vi "Get Initial FP Control Positions.vi"(8 "error in (no error)":errorcluster, 9 "Pane 2":refnum<vi>, 10 "Pane":refnum<vi>, 11 "Message Log in":refnum<class "Message Log.lvclass">) -> (0 "error out":errorcluster, 3 "Message Log out":refnum<class "Message Log.lvclass">)   [LabVIEW 2017, in "Message Log.lvclass"]
doc: "Get the initial positons of resizable front panel elements"
uses:
  Message Log.lvclass
  Message Log.lvclass/Message Log.ctl
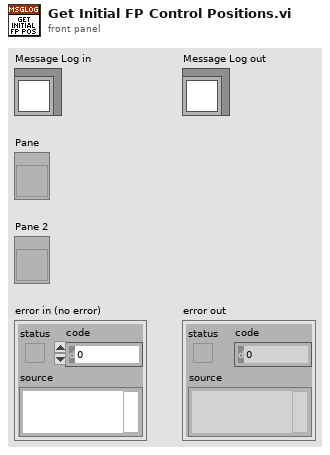
[diagram p1: front panel]
types:
  T1 = typedef "LVBoundsTypeDef.ctl" = cluster{"Width":u32, "Height":u32}
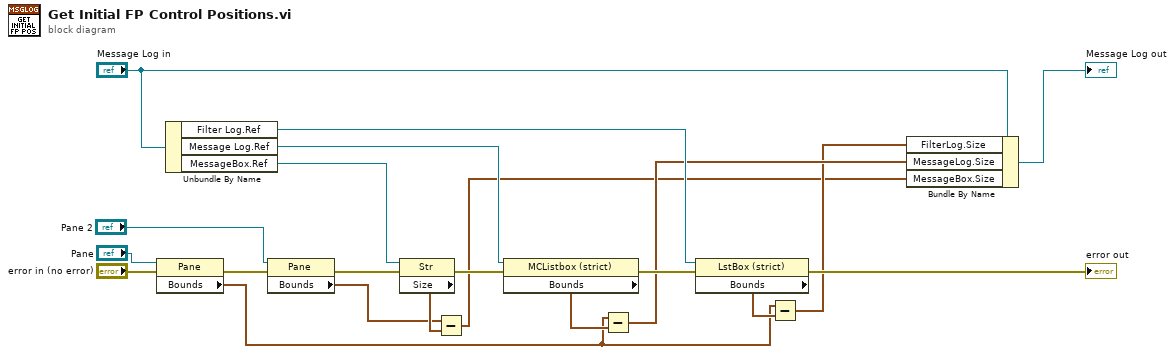
[diagram p0: block diagram]
diagram:
  n1 = property class="Pane"(reference="Pane", error in="error in (no error)") -> (error out=w14:errorcluster, "Bounds"=w1:T1)  [unwired: 1 out]
  n2 = Unbundle By Name("Message Log in") -> ("Filter Log.Ref"=w12:refnum<vi>, "Message Log.Ref"=w15:refnum<vi>, "MessageBox.Ref"=w8:refnum<vi>)
  n3 = property class="Pane"(reference="Pane 2", error in=w14) -> (error out=w7:errorcluster, "Bounds"=w6:T1)  [unwired: 1 out]
  n4 = property class="Str"(reference=w8, error in=w7) -> (error out=w5:errorcluster, "Size"=w9:T1)  [unwired: 1 out]
  n5 = Subtract(x=w6, y=w9) -> (x-y=w2:T1)
  n6 = property class="MCListbox (strict)"(reference=w15, error in=w5) -> (error out=w13:errorcluster, "Bounds"=w16:T1)  [unwired: 1 out]
  n7 = Subtract(x=w1, y=w16) -> (x-y=w4:T1)
  n8 = property class="LstBox (strict)"(reference=w12, error in=w13) -> (error out=→"error out":errorcluster, "Bounds"=w21:T1)  [unwired: 1 out]
  n9 = Subtract(x=w1, y=w21) -> (x-y=w3:T1)
  n10 = Bundle By Name(cluster="Message Log in", "FilterLog.Size"=w3, "MessageLog.Size"=w4, "MessageBox.Size"=w2) -> (→"Message Log out":refnum<class "Message Log.lvclass">)
